vi "fpga_transmission_control_3V13.vi"() -> ()   [LabVIEW 2017]
uses:
  Control 1.ctl
  <vilib>/Platform/TimedLoop/XDataNode/timing_clust.ctl
  <vilib>/Platform/TimedLoop/XDataNode/nitl_modes.ctl
  <vilib>/Platform/TimedLoop/XDataNode/wakeup.ctl
  <vilib>/Instr/_visa.llb/VISA Configure Serial Port (Serial Instr).vi
  <vilib>/platform/TimedLoop/XDataNode/XDataNode.xnode
  <vilib>/Platform/TimedLoop/XDataNode/XDNodeRunTimeDep.lvlib
panel:
  out "Complete Time":u32
  out "Timer":u32
  out "Output":bool
  out "outcome":u32
  out "currentType":string
  out "Time":dbl(slide) scale=0.0..100.0
  out "Progress":dbl(slide) scale=0.0..100.0
  in  "error in (no error)":errorcluster
  out "PWM":bool
  out "pattern":u32
  in  "Timeslot":bool
  out "type":string
  out "Kombi Chart":cluster{u16, i16}(graph)
  out "contingency":string
  in  "Array":T2(array[cluster]) {"duration" step=1}
  out "Timeslot":i32
  out "Sign":bool
  out "deleted portion":u8[](array[numeric])
  out "data":bool
  out "x-y":u16
  out "Error String":string
  out "error out":errorcluster
  out "Timing":u32
  out "Int_pixel":i16
  out "Pixel":u16(graph)
  out "AD_Value":i16
  in  "millisecond timer value 2":u32
  out "AD_Chart":i16(graph)
  in  "Path":path
  out "Read":bool
  in  "Stop Program":bool
  in  "Start":bool
  in  "VISA resource name":refnum<visa-resource-name>
  # "UR Elektronik Biologie\nTerminal V 3.8"
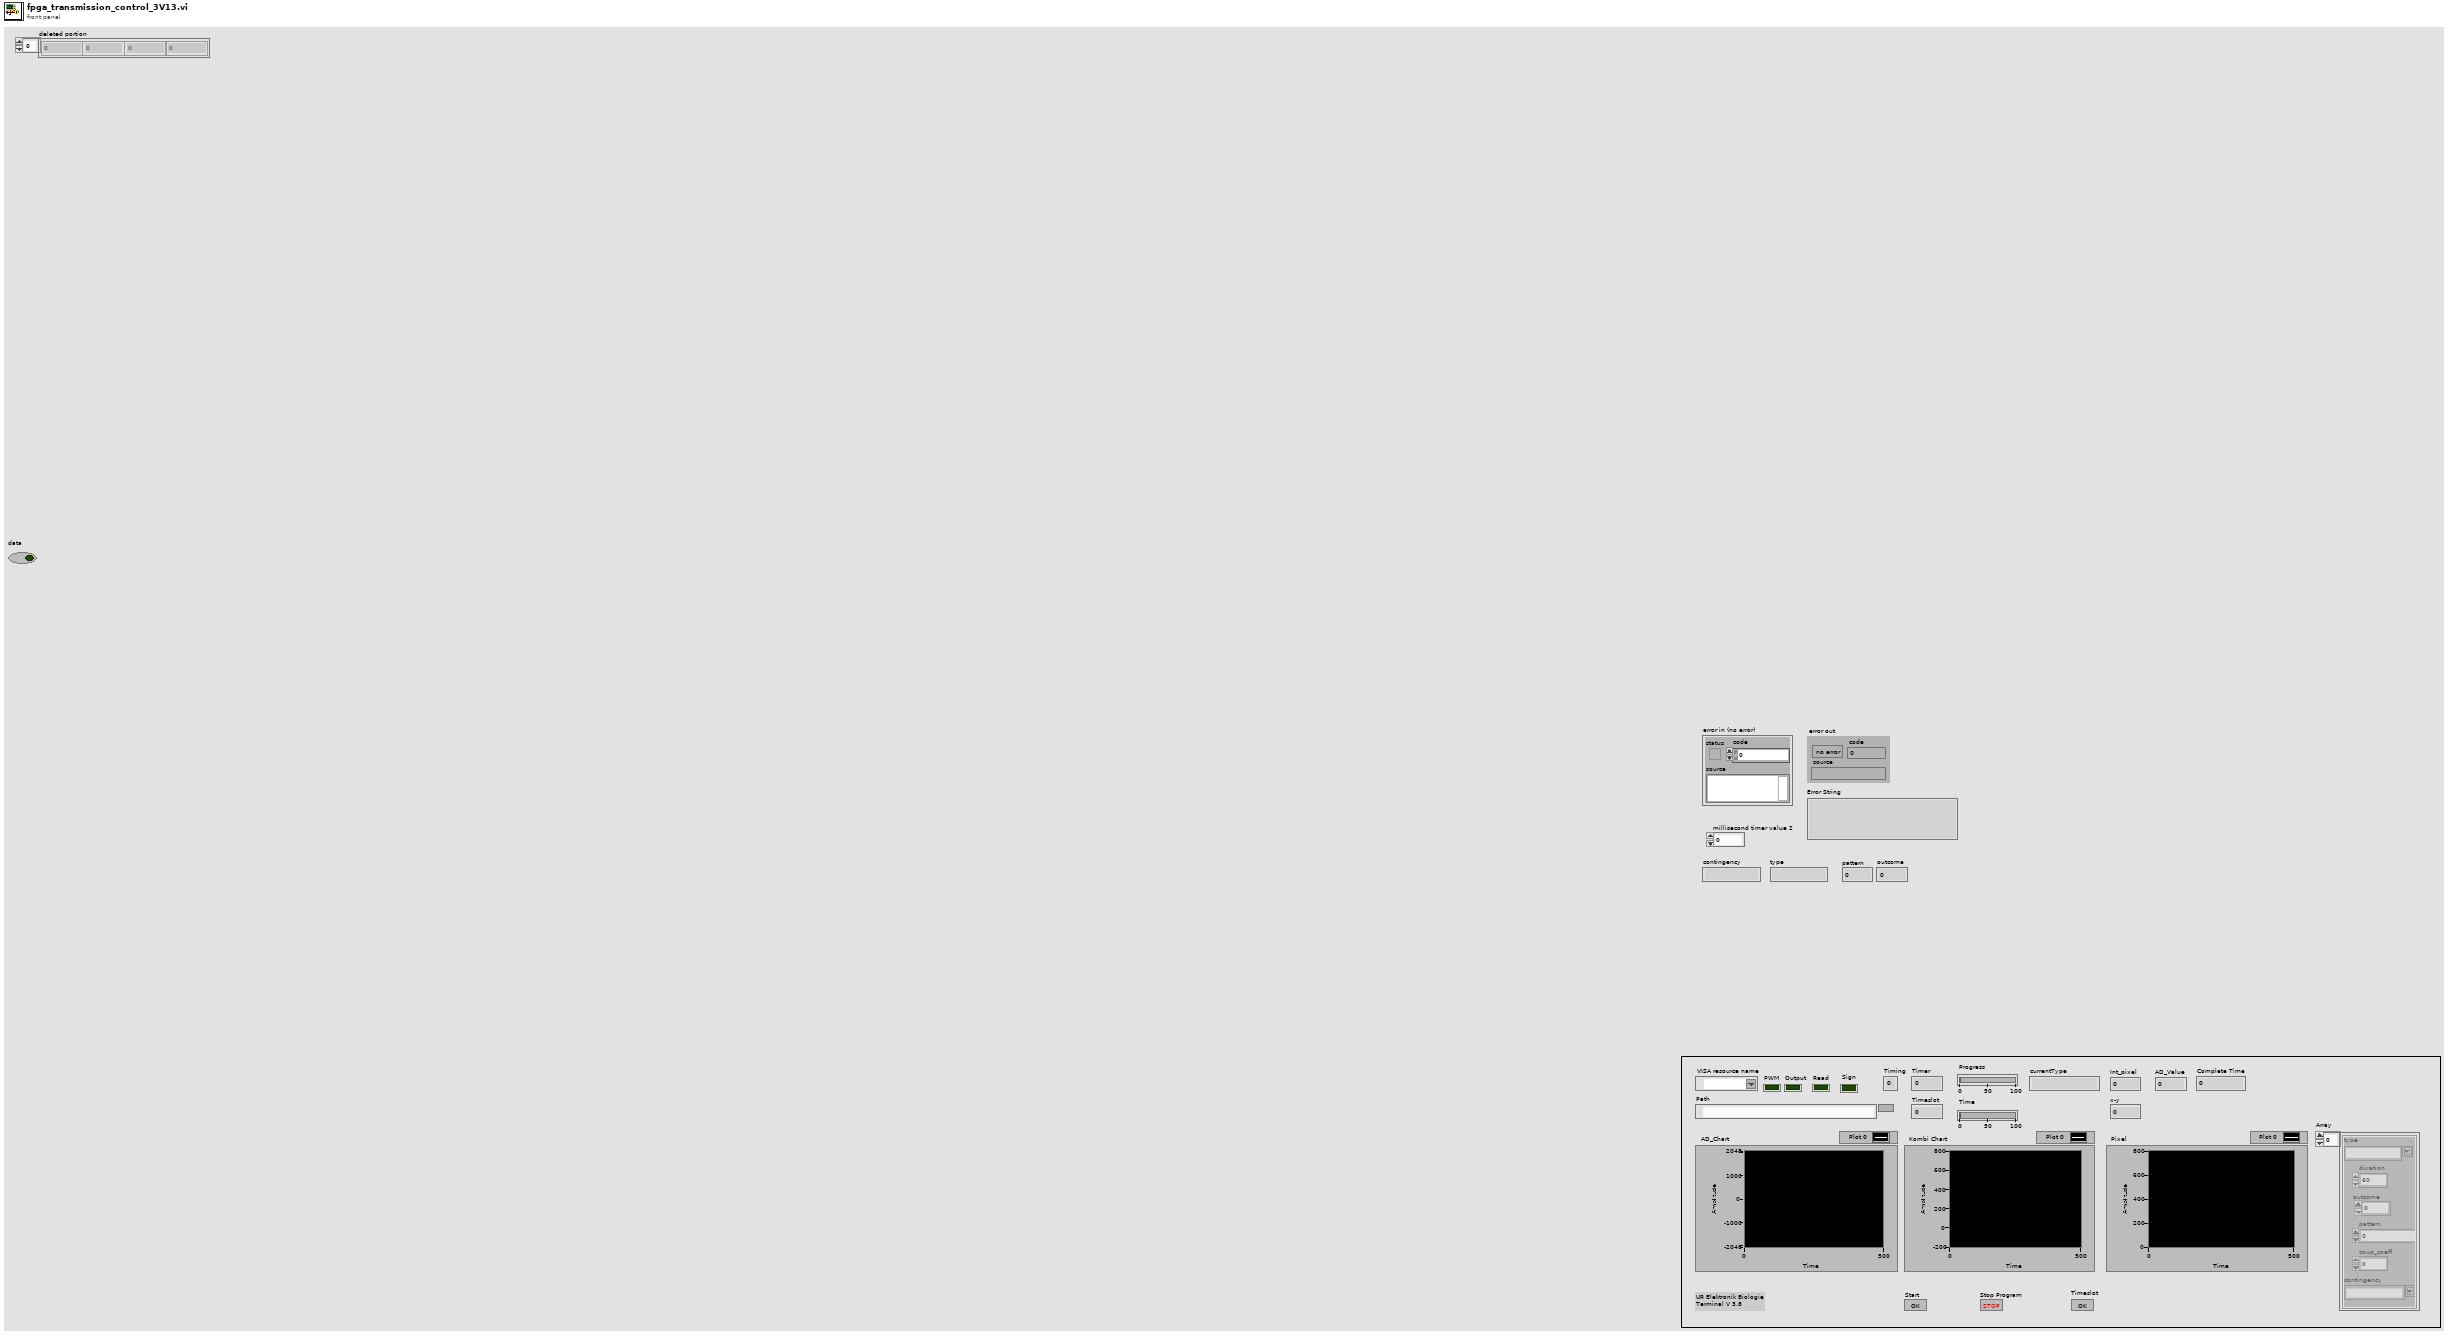
[diagram p1: front panel]
types:
  T1 = typedef "Control 1.ctl" = u32
  T2 = cluster{"type":string, "duration":T1, "outcome":u32, "pattern":u32, "coup_coeff":u32, "contingency":string}[]
  T3 = typedef "XDNodeRunTimeDep.lvlib/timing_clust.ctl" = cluster{"Expected End [f-1]":u64, "Actual End [f-1]":u64, "Finished Late? [f-1]":bool, "Expected End [i-1]":u64, "Actual End [i-1]":u64, "Finished Late? [i-1]":bool, "Expected Start [i]":u64, "Actual Start [i]":u64, "Expected Start [f]":u64, "Actual Start [f]":u64, "Source Name":string, "Structure Name":string, "Period":i64, "Deadline":i64, "Offset":i64, "Start":i64, "Priority":i32, "Timeout":i32, "Mode":T4, "Wakeup Reason":T5, "Error":errorcluster, "Source Type":string, "Secondary Source Type":string, "Global End Time":u64, "Global Start Time":u64, "Frame Duration":u64, "Iteration Duration":u64, "Assigned CPU":i32, "I/O Scan Engine Mode":u32}
  T4 = typedef "XDNodeRunTimeDep.lvlib/nitl_modes.ctl" = enum32{"No Change", "Process missed periods, maintain original phase", "Discard missed periods, maintain original phase", "Process missed periods, ignore original phase", "Discard missed periods, ignore original phase"}
  T5 = typedef "XDNodeRunTimeDep.lvlib/wakeup.ctl" = enum32{"Normal", "Aborted", "Asynchronous wakeup", "Timing source error", "Timed loop error", "Timeout"}
  T6 = cluster{"String":string, i32, i32, u32, u32, "String":string}[]
  T7 = cluster{"type":string, "duration":T1, "outcome":u32, "pattern":u32, "coup_coeff":u32, "contingency":string}
  T8 = enum16{"Idel", "State1", "State2", "State3", "State4"}
  T9 = enum16{"open", "replace", "create", "open or create", "replace or create", "replace or create with confirmation"}
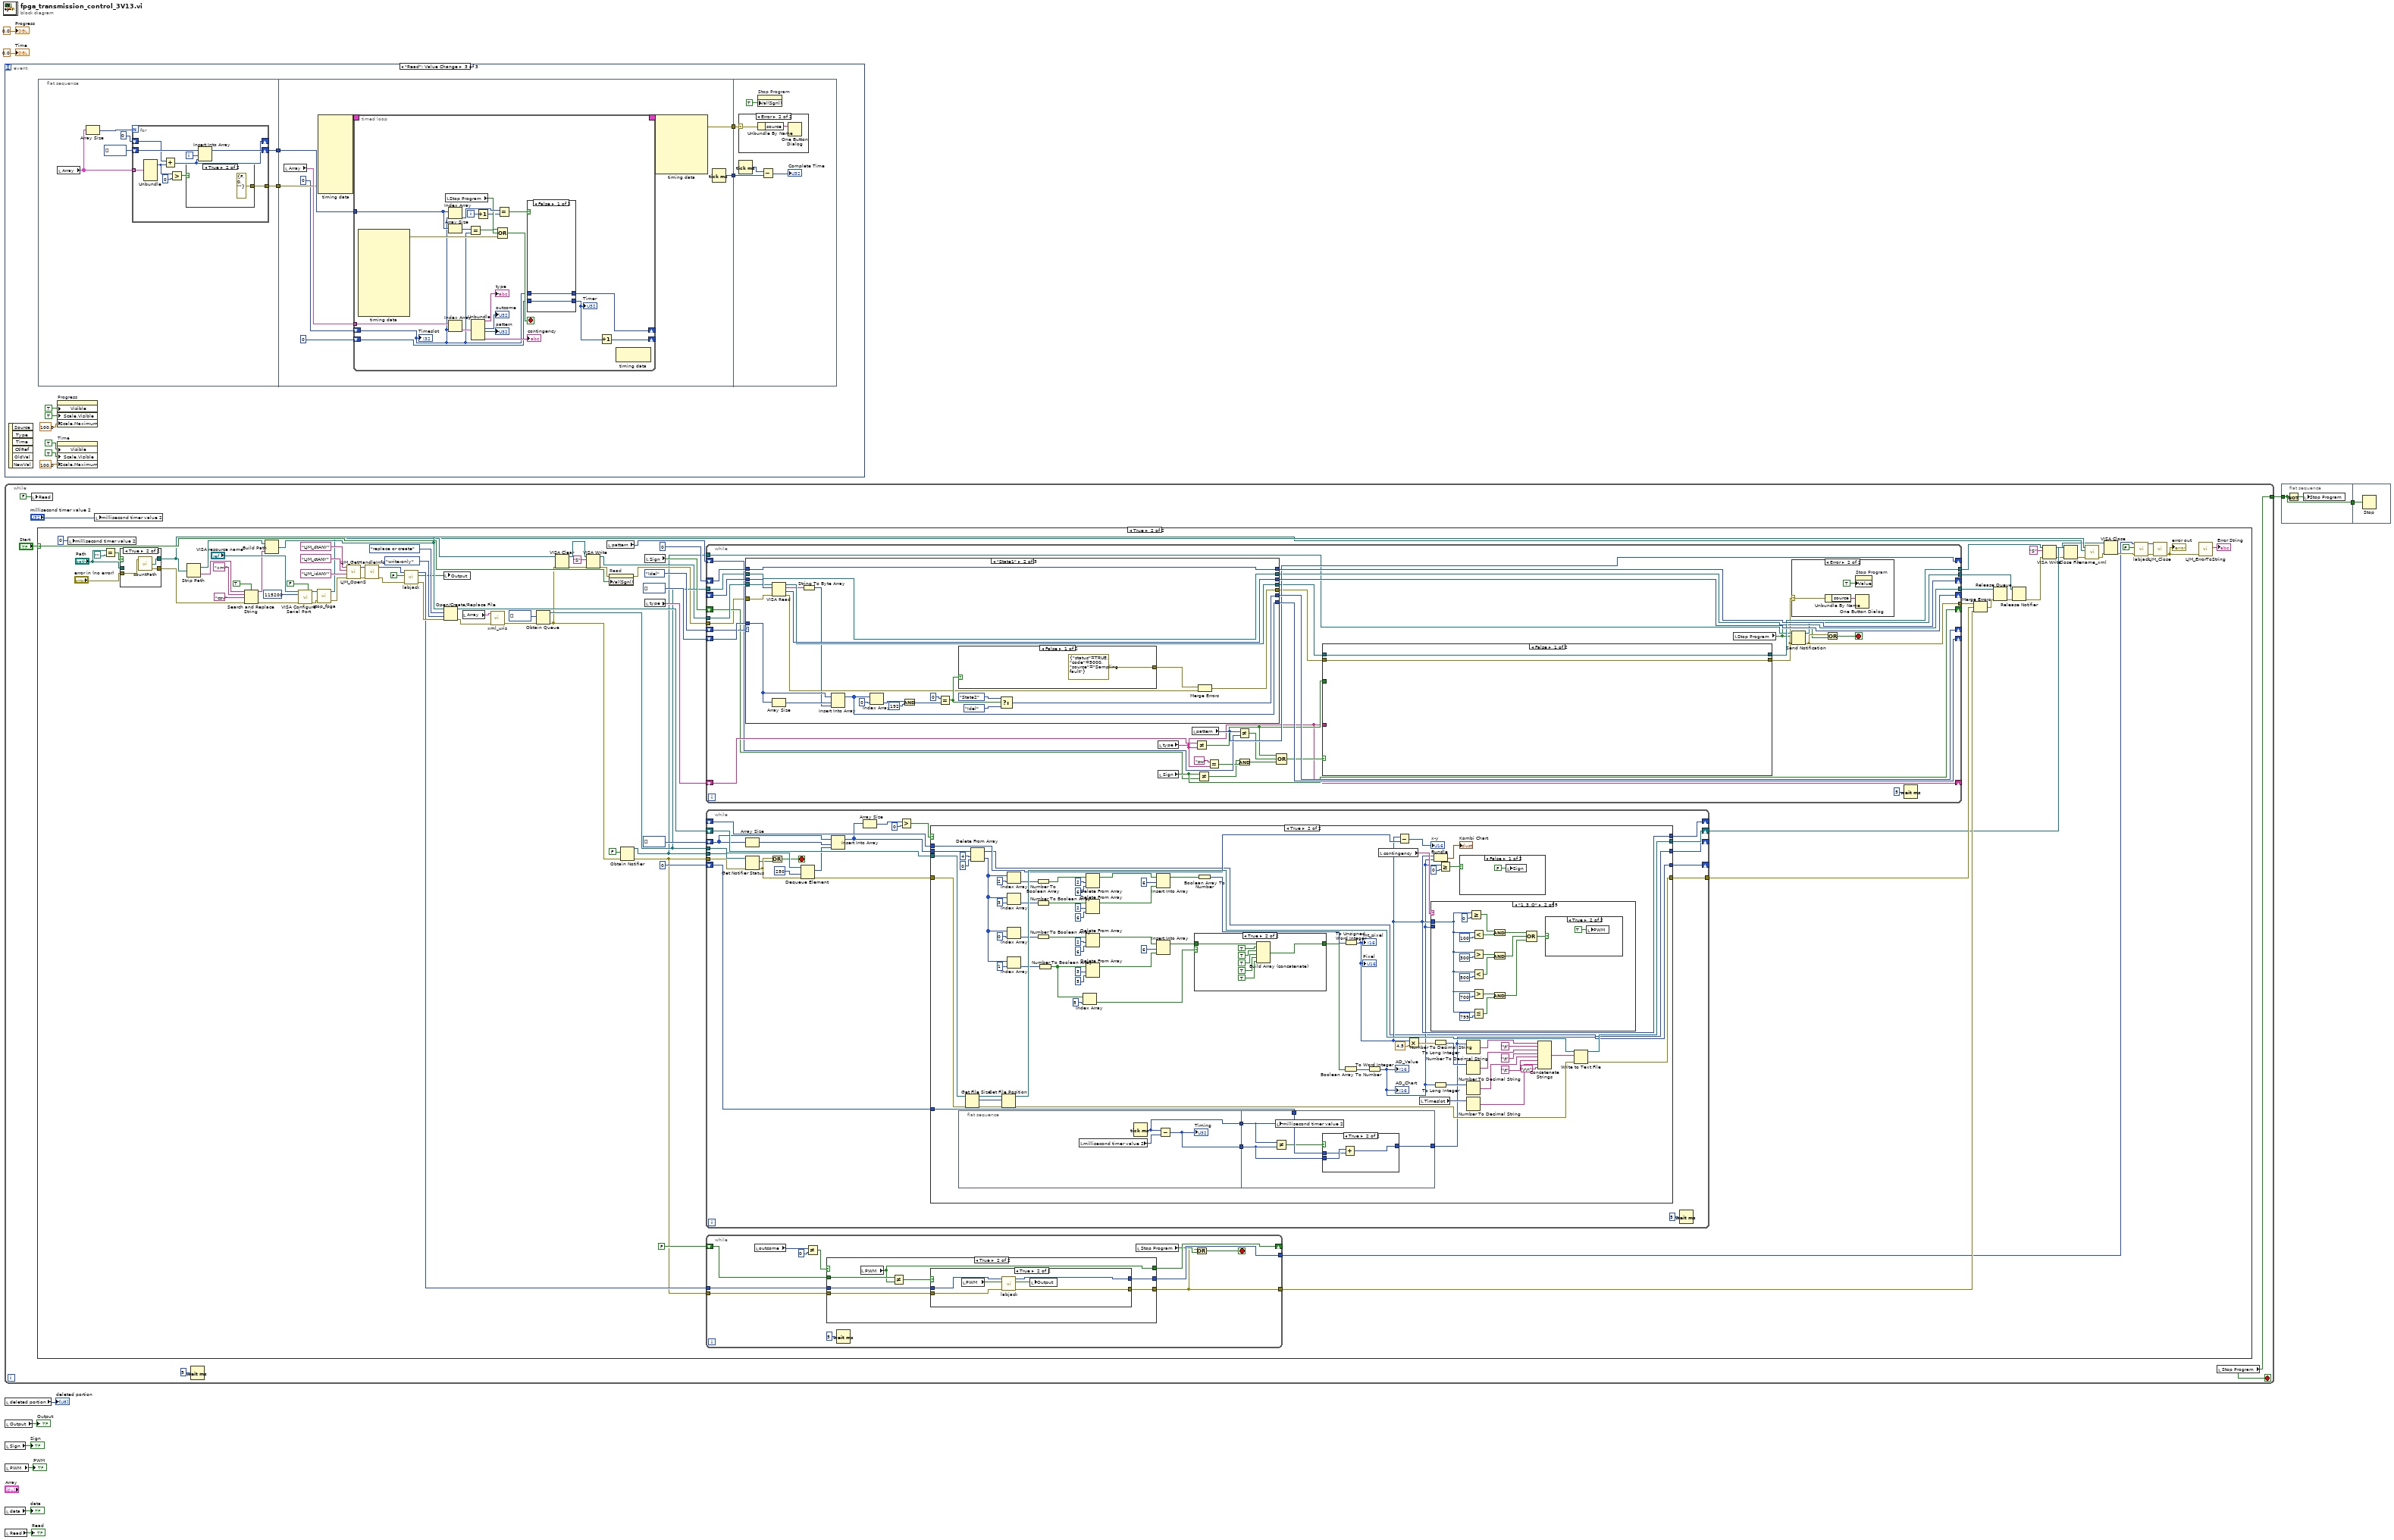
[diagram p0: block diagram]
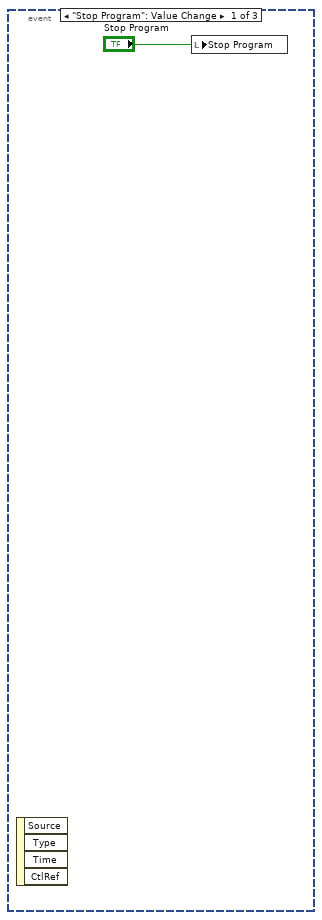
[diagram p2: hidden frame]
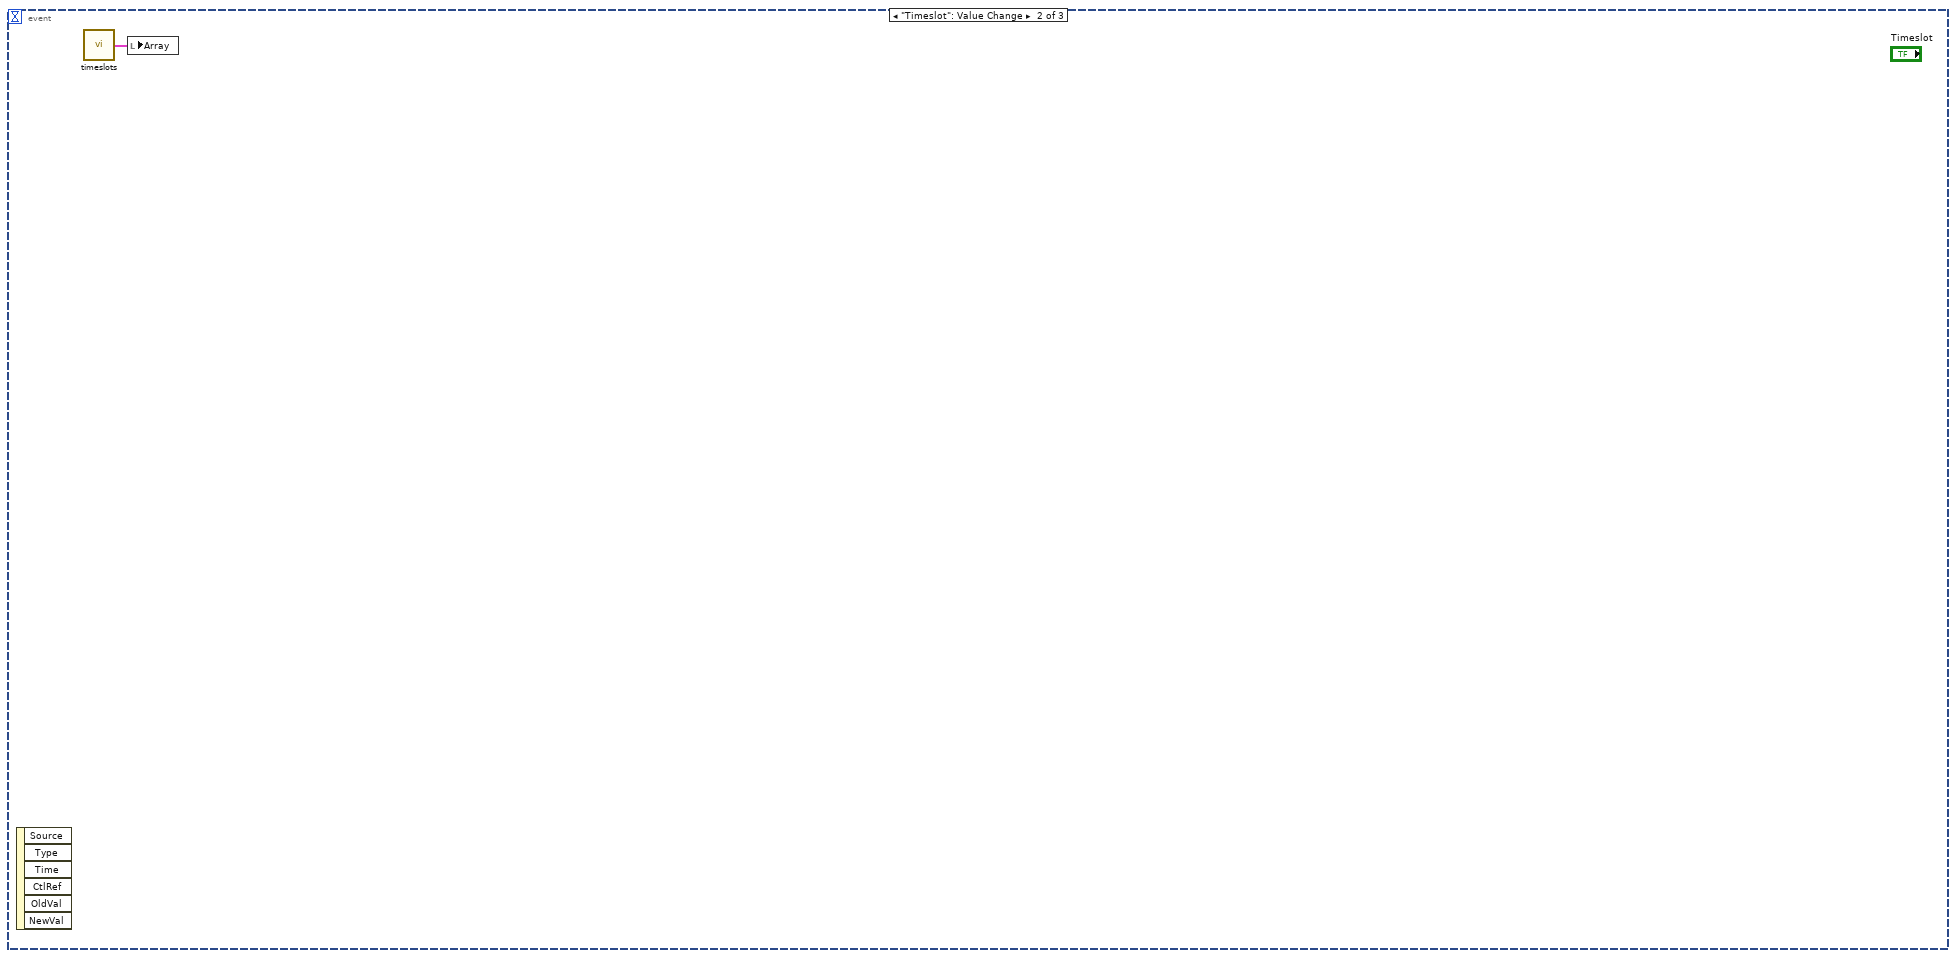
[diagram p3: hidden frame]
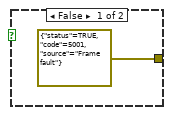
[diagram p4: hidden frame]
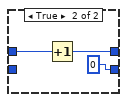
[diagram p5: hidden frame]
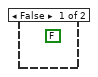
[diagram p7: hidden frame]
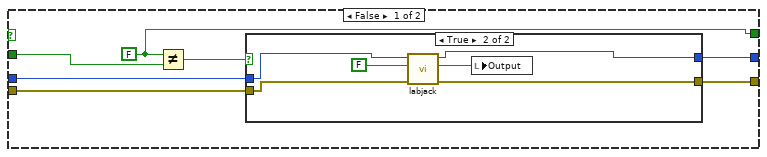
[diagram p9: hidden frame]
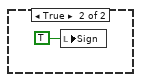
[diagram p13: hidden frame]
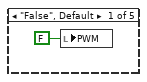
[diagram p14: hidden frame]
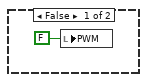
[diagram p15: hidden frame]
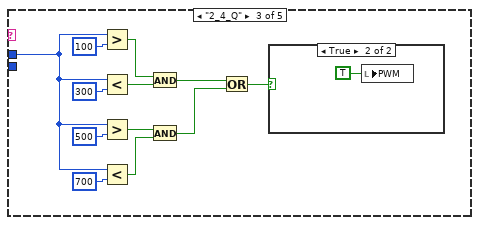
[diagram p16: hidden frame]
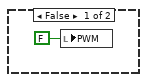
[diagram p17: hidden frame]
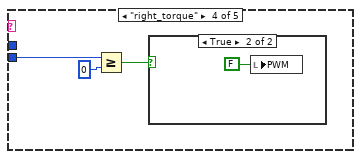
[diagram p18: hidden frame]
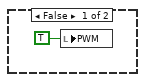
[diagram p19: hidden frame]
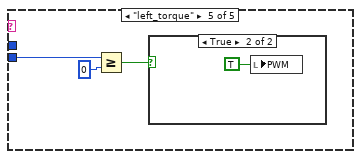
[diagram p20: hidden frame]
diagram:
  n1 = event shown="[2] \"Read\": Value Change" {
    selector: _ -> [_ _ _]
    dyn-events: _ -> [_ _ _]
    timeout: _ -> [_ _ _]
    event "Stop Program": Value Change {
      n2 = event-data() -> ()  [unwired: 1 in, 4 out]
      n3 = local write "Stop Program"("Stop Program") -> ()
    }
    event "Timeslot": Value Change {
      n4 = event-data() -> ()  [unwired: 1 in, 6 out]
      n5 = call "timeslots.vi"() -> ("array of clusters"=w12:T6)  [unwired: 1 in, 1 out]
      n6 = local write "Array"(w12) -> ()
    }
    event "Read": Value Change {
      n7 = event-data() -> ()  [unwired: 1 in, 6 out]
      n8 = flat-sequence {
        tunnel: [w24] -> w16
        tunnel: [w23] -> w15
        tunnel: w16 -> [w46]
        tunnel: w15 -> [w45]
        tunnel: [w44] -> w14
        tunnel: [w42] -> w13
        tunnel: w14 -> [w87]
        tunnel: w13 -> [w84]
        frame #0 {
          n9 = local read "Array"() -> (w27:T2)
          n10 = Array Size(array=w27) -> (size(s)=w28:i32)
          n11 = for {
            N: w28 -> [_]
            tunnel: w27 -> [w38] mode=indexing
            shift-right: [w36] -> w24
            shift-left: T1[] [] -> [w35]
            shift-right: [w33] -> _
            shift-left: T1 0 ("duration") -> [w34]
            tunnel: [w29] -> w23
            i -> [w37]
            n12 = Unbundle(w38) -> ("duration"=w31:T1)  [unwired: 5 out]
            n13 = Add(x=w34, y=w31) -> (x+y=w33:T1)
            n14 = Greater?(x=w31, y=T1 0) -> (0:w32:bool)
            n15 = case shown="True" w32 {
              tunnel: [errorcluster {"status"=TRUE, "code"=5001, "source"="Frame fault"} ("error constant") errorcluster {"status"=FALSE, "code"=0, "source"=""} ("error constant")] -> w29
              frame False {
              }
              frame True {
              }
            }
            n16 = Insert Into Array(array=w35, index=w37, new element=w33) -> (w36:T1[])
          }
        }
        frame #1 {
          n17 = local read "Array"() -> (w47:T2)
          n18 = node-c288(w45) -> (w49:T3)  [unwired: 9 in]
          n19 = timed-loop {
            timing: w49 -> [_]
            timing-out: [_] -> w48
            tunnel: w47 -> [w65]
            tunnel: w46 -> [w59]
            shift-right: [w62] -> _
            shift-left: T1 0 ("duration") -> [w57]
            shift-right: [w52] -> _
            shift-left: 0 -> [w51]
            i -> [w54]
            stop <- w64 stop-if-true
            n20 = node-c288() -> (w63:errorcluster)  [unwired: 1 in, 11 out]
            n21 = local read "Stop Program"() -> (w56:bool)
            n22 = Index Array(array=w59, index=w57) -> (element=w61:T1)
            n23 = Array Size(array=w59) -> (size(s)=w58:i32)
            n24 = Index Array(array=w65, index=w57) -> (element=w70:T7)
            n25 = Equal?(x=w58, y=w57) -> (x = y?=w55:bool)
            n26 = Unbundle(w70) -> ("type"=→"type":string, "outcome"=→"outcome":u32, "pattern"=→"pattern":u32, "contingency"=→"contingency":string)  [unwired: 2 out]
            n27 = Increment(x=w54) -> (x+1=w53:i32)
            n28 = Equal?(x=w61, y=w53) -> (x = y?=w60:bool)
            n29 = Compound Arithmetic op=OR(w56, w55, w63) -> (w64:bool)
            n30 = case shown="False" w60 {
              tunnel: [w72 w75] -> w62
              tunnel: w57 -> [w72 w74]
              tunnel: w51 -> [w71 _]
              tunnel: [w71 0] -> w50
              frame False {
              }
              frame True {
                n31 = Increment(x=w74) -> (x+1=w75:T1)
              }
            }
            "Timer" <- w50
            n32 = Increment(x=w50) -> (x+1=w52:i32)
            n33 = node-c288() -> ()  [unwired: 1 in, 1 out]
            "Timeslot" <- w57
          }
          n34 = node-c288(w48) -> (w44:errorcluster)  [unwired: 6 out]
          n35 = Tick Count (ms)() -> (millisecond timer value=w42:u32)
        }
        frame #2 {
          n36 = case shown="Error" w87 {
            selector: w87 -> [_ w90]
            frame No Error {
            }
            frame Error {
              n37 = Unbundle By Name(w90) -> ("source"=w89:string)
              n38 = One Button Dialog(message=w89) -> ()  [unwired: 1 in, 1 out]
            }
          }
          n39 = Tick Count (ms)() -> (millisecond timer value=w85:u32)
          n40 = property on="Stop Program" class="Bool (strict)"("Val(Sgnl)"=TRUE) -> ()  [unwired: 2 in, 2 out]
          n41 = Subtract(x=w85, y=w84) -> (x-y=→"Complete Time":u32)
        }
      }
      n42 = property on="Progress" class="Slide (strict)"("Visible"=TRUE, "Scale.Visible"=TRUE ("Visible"), "Scale.Maximum"=100.0 ("Scale.Range:Maximum")) -> ()  [unwired: 2 in, 2 out]
      n43 = property on="Time" class="Slide (strict)"("Visible"=TRUE, "Scale.Visible"=TRUE ("Visible"), "Scale.Maximum"=100.0 ("Scale.Range:Maximum")) -> ()  [unwired: 2 in, 2 out]
    }
  }
  n44 = while {
    tunnel: [w94] -> w10
    stop <- w94 stop-if-true
    n45 = local write "Read"(FALSE) -> ()
    n46 = case shown="True" "Start" {
      selector: "Start" -> [_ w172]
      frame False {
        (unwired) FALSE
      }
      frame True {
        n47 = local write "millisecond timer value 2"(u32 0 ("millisecond timer value 2")) -> ()
        n48 = Equal?(x="Path", y=path "") -> (x = y?=w159:bool)
        n49 = case shown="True" w159 {
          tunnel: [w180 w183] -> w125
          tunnel: "Path" -> [w180 _]
          tunnel: [w179 w182] -> w134
          tunnel: "error in (no error)" -> [w179 w181]
          frame False {
          }
          frame True {
            n50 = call "countPath.vi"("error in (no error)"=w181) -> ("error out"=w182:errorcluster, "appended path"=w183:path)
          }
        }
        n51 = Strip Path(path=w125) -> (stripped path=w138:path, name=w137:string)
        n52 = Search and Replace String(case sensitive?=TRUE ("ignore case? (F)"), input string=w137, search string="xml", replace string="csv" ("replace string (\"\")"), error in=w134) -> (result string=w131:string, error out=w133:errorcluster)  [unwired: 3 in, 2 out]
        n53 = Build Path(base path=w138, name or relative path=w131) -> (appended path=w126:path)
        n54 = call-poly "VISA Configure Serial Port"("VISA resource name"="VISA resource name", "Enable Termination\nChar (T)"=FALSE ("Enable Termination\nChar (T)"), "baud rate (9600)"=u32 115200, "error in (no error)"=w133) -> ("VISA resource name out"=w118:refnum<visa-resource-name>, "error out"=w117:errorcluster)  [unwired: 10 in]
        n55 = call "stop_fpga.vi"("error in (no error)"=w117, "reference"=w118) -> ("error out"=w116:errorcluster, "VISA resource name out"=w109:refnum<visa-resource-name>)  [unwired: 2 in]
        n56 = call "LJM_OpenS.vi"("error in"=w116, "Identifier"="LJM_idANY", "ConnectionType"="LJM_ctANY", "DeviceType"="LJM_dtANY") -> ("error out"=w162:errorcluster, "Handle"=w161:i32)  [unwired: 6 in]
        n57 = call "LJM_GetHandleInfo.vi"("error in"=w162, "Handle In"=w161) -> ("error out"=w164:errorcluster, "Handle Out"=w163:i32)  [unwired: 2 in, 6 out]
        n58 = call "labjack.vi"("error out"=w164, "Boolean"=FALSE, "Handle Out"=w163) -> ("error out 2"=w167:errorcluster, "Boolean 2"=w124:bool, "Handle Out 2"=w166:i32)  [unwired: 6 in]
        n59 = local write "Output"(w124) -> ()
        n60 = Open/Create/Replace File(file path (use dialog)=w126, error in=w167, operation (0:open)=T9."replace or create", access (0:read/write)=enum16{"read/write", "read-only", "write-only"}."write-only") -> (refnum out=w141:refnum<file>, error out=w139:errorcluster)  [unwired: 2 in, 1 out]
        n61 = local read "Array"() -> (w140:T2)
        n62 = call "xml_uris.vi"("error in"=w139, "Array"=w140) -> ("error out"=w110:errorcluster)  [unwired: 2 in, 2 out]
        n63 = Obtain Queue(element data type=u8[] [], error in (no error)=w110) -> (queue out=w112:refnum<queue>, error out=w97:errorcluster)  [unwired: 3 in, 1 out]
        n64 = VISA Clear(VISA resource name=w109, error in (no error)=w97) -> (VISA resource name out=w108:refnum<visa-resource-name>, error out=w106:errorcluster)
        n65 = VISA Write(VISA resource name=w108, write buffer="S", error in (no error)=w106) -> (VISA resource name out=w107:refnum<visa-resource-name>, error out=w115:errorcluster)  [unwired: 1 out]
        n66 = local read "pattern"() -> (w144:u32)
        n67 = property on="Read" class="Bool (strict)"(error in=w115, "Val(Sgnl)"=w172) -> (error out=w105:errorcluster)  [unwired: 1 in, 1 out]
        n68 = Obtain Notifier(notification data type=FALSE, error in (no error)=w97) -> (notifier out=w103:refnum<notifier>, error out=w96:errorcluster)  [unwired: 2 in, 1 out]
        n69 = local read "Sign"() -> (w143:bool)
        n70 = local read "type"() -> (w168:string)
        n71 = while {
          tunnel: w107 -> [w428]
          shift-right: [w422] -> _
          shift-left: u8[] [] -> [w427]
          tunnel: [w404] -> w121
          shift-right: [w426] -> _
          shift-left: T8."Idel" -> [w425]
          shift-right: [w424] -> _
          shift-left: _ -> [w423]
          shift-right: [w421] -> _
          shift-left: u8 0 -> [w420]
          shift-right: [w411] -> _
          shift-left: w168 -> [w419]
          shift-right: [w418] -> _
          shift-left: w144 -> [w417]
          shift-right: [w416] -> _
          shift-left: w143 -> [w415]
          tunnel: w112 -> [w403]
          tunnel: [w402] -> w111
          tunnel: w103 -> [w399]
          tunnel: w105 -> [w400]
          tunnel: [w396] -> w100
          tunnel: [w397] -> w101
          stop <- w394 stop-if-true
          n72 = case shown="\"State1\"" w425 {
            tunnel: w428 -> [w546 w573 w591]
            tunnel: w400 -> [w547 w574 w585]
            tunnel: w427 -> [w550 w576 w598]
            tunnel: [w554 w577 w591] -> w405
            tunnel: [w553 w562 w584] -> w406
            tunnel: [w555 w575 w594] -> w426
            tunnel: [w552 w578 w592] -> w424
            tunnel: w423 -> [_ w579 w592]
            tunnel: [w550 w572 w597] -> w422
            tunnel: [w549 w571 u8 0] -> w421
            tunnel: w420 -> [w549 w571 _]
            tunnel: w403 -> [w544 w565 w587]
            tunnel: [w544 w565 w586] -> w402
            frame "Idel", Default {
              n73 = local write "data"(FALSE ("data")) -> ()
              n74 = property class="Serial Instr"(reference=w546, error in=w547) -> (reference out=w554:refnum<visa-resource-name>, error out=w553:errorcluster, "Serial Settings:Number of Bytes at Serial Port"=w552:u32)
              n75 = Greater Or Equal?(x=w552, y=u8 4) -> (x >= y?=w545:bool)
              n76 = Select(t=T8."State1", s=w545, f=T8."Idel") -> (s? t:f=w555:T8)
            }
            frame "State1" {
              n77 = VISA Read(VISA resource name=w573, byte count=w579, error in (no error)=w574) -> (VISA resource name out=w577:refnum<visa-resource-name>, read buffer=w559:string, return count=w578:u32, error out=w560:errorcluster)
              n78 = Array Size(array=w576) -> (size(s)=w564:i32)
              n79 = String To Byte Array(string=w559) -> (unsigned byte array=w558:u8[])
              n80 = Insert Into Array(array=w576, index=w564, new element=w558) -> (w572:u8[])
              n81 = Index Array(array=w572, index=0) -> (element=w569:u8)
              n82 = And(x=w569, y=u8 192) -> (x .and. y?=w568:u8)
              n83 = Equal?(x=u8 0, y=w568) -> (x = y?=w561:bool)
              n84 = case shown="False" w561 {
                tunnel: [errorcluster {"status"=TRUE, "code"=5000, "source"="Sampling fault"} ("error constant") errorcluster {"status"=FALSE, "code"=0, "source"=""} ("error constant")] -> w563
                frame False {
                }
                frame True {
                }
              }
              n85 = Select(t=T8."State2", s=w561, f=T8."Idel") -> (s? t:f=w575:T8)
              n86 = Merge Errors(w563, w560) -> (w562:errorcluster)
            }
            frame "State2" {
              n87 = Delete From Array(array=w598, length=4, index=0) -> (deleted portion=w588:u8[], array with subset deleted=w597:u8[])
              n88 = Array Size(array=w597) -> (size(s)=w596:i32)
              n89 = Enqueue Element(queue=w587, element=w588, error in (no error)=w585) -> (queue out=w586:refnum<queue>, error out=w584:errorcluster)  [unwired: 1 in, 1 out]
              n90 = Greater Or Equal?(x=w596, y=4) -> (x >= y?=w589:bool)
              n91 = Select(t=T8."State2", s=w589, f=T8."Idel") -> (s? t:f=w594:T8)
            }
          }
          n92 = local read "type"() -> (w411:string)
          n93 = local read "Sign"() -> (w416:bool)
          n94 = local read "pattern"() -> (w418:u32)
          n95 = Not Equal?(x=w419, y=w411) -> (x != y?=w412:bool)
          n96 = Not Equal?(x=w416, y=w415) -> (x != y?=w408:bool)
          n97 = Equal?(x="sw", y=w411) -> (x = y?=w409:bool)
          n98 = Not Equal?(x=w418, y=w417) -> (x != y?=w414:bool)
          n99 = And(x=w408, y=w409) -> (x .and. y?=w407:bool)
          n100 = Compound Arithmetic op=OR(w412, w414, w407) -> (w413:bool)
          n101 = case shown="False" w413 {
            tunnel: w405 -> [w433 w437]
            tunnel: [w433 w440] -> w404
            tunnel: w406 -> [w432 w436]
            tunnel: [w432 w441] -> w398
            tunnel: w411 -> [_ w434]
            tunnel: w412 -> [_ w435]
            frame False {
            }
            frame True {
              n102 = case shown="True" w435 {
                tunnel: [w443 w449] -> w439
                tunnel: [w444 w448] -> w438
                tunnel: w437 -> [w444 w446]
                tunnel: w436 -> [w443 w445]
                frame False {
                }
                frame True {
                  n103 = VISA Write(VISA resource name=w446, write buffer="1W", error in (no error)=w445) -> (VISA resource name out=w448:refnum<visa-resource-name>, error out=w449:errorcluster)  [unwired: 1 out]
                }
              }
              n104 = case shown="\"fs\"" w434 {
                tunnel: w438 -> [w451 w458 w463 w471 w482 w519]
                tunnel: [w453 w457 w462 w465 w481 w518] -> w440
                tunnel: w439 -> [w450 w456 w461 w470 w484 w521]
                tunnel: [w452 w455 w460 w466 w483 w520] -> w442
                frame "False", Default {
                  n105 = VISA Write(VISA resource name=w451, write buffer="s4s", error in (no error)=w450) -> (VISA resource name out=w453:refnum<visa-resource-name>, error out=w452:errorcluster)  [unwired: 1 out]
                }
                frame "optomotorR" {
                  n106 = VISA Write(VISA resource name=w458, write buffer="s3r", error in (no error)=w456) -> (VISA resource name out=w457:refnum<visa-resource-name>, error out=w455:errorcluster)  [unwired: 1 out]
                }
                frame "optomotorL" {
                  n107 = VISA Write(VISA resource name=w463, write buffer="s3l", error in (no error)=w461) -> (VISA resource name out=w462:refnum<visa-resource-name>, error out=w460:errorcluster)  [unwired: 1 out]
                }
                frame "yt" {
                  n108 = local read "pattern"() -> (w469:u32)
                  n109 = VISA Write(VISA resource name=w471, write buffer="s1s", error in (no error)=w470) -> (VISA resource name out=w468:refnum<visa-resource-name>, error out=w467:errorcluster)  [unwired: 1 out]
                  n110 = case shown="9" w469 {
                    tunnel: w468 -> [w474 w478]
                    tunnel: w467 -> [w473 w477]
                    tunnel: [w473 w476] -> w466
                    tunnel: [w474 w475] -> w465
                    frame 0, Default {
                    }
                    frame 9 {
                      n111 = VISA Write(VISA resource name=w478, write buffer="D", error in (no error)=w477) -> (VISA resource name out=w475:refnum<visa-resource-name>, error out=w476:errorcluster)  [unwired: 1 out]
                    }
                  }
                }
                frame "sw" {
                  n112 = local read "pattern"() -> (w480:u32)
                  n113 = case shown="7" w480 {
                    tunnel: w484 -> [w485 w490 w506]
                    tunnel: [w485 w488 w505] -> w483
                    tunnel: w482 -> [w486 w491 w504]
                    tunnel: [w486 w489 w503] -> w481
                    frame 0, Default {
                    }
                    frame 8 {
                      n114 = local read "Sign"() -> (w487:bool)
                      n115 = case shown="False" w487 {
                        tunnel: w490 -> [w493 w500]
                        tunnel: [w492 w499] -> w488
                        tunnel: w491 -> [w495 w498]
                        tunnel: [w494 w497] -> w489
                        frame True {
                          n116 = VISA Write(VISA resource name=w495, write buffer="G", error in (no error)=w493) -> (VISA resource name out=w494:refnum<visa-resource-name>, error out=w492:errorcluster)  [unwired: 1 out]
                        }
                        frame False {
                          n117 = VISA Write(VISA resource name=w498, write buffer="B", error in (no error)=w500) -> (VISA resource name out=w497:refnum<visa-resource-name>, error out=w499:errorcluster)  [unwired: 1 out]
                        }
                      }
                    }
                    frame 7 {
                      n118 = local read "Sign"() -> (w502:bool)
                      n119 = case shown="True" w502 {
                        tunnel: w506 -> [w508 w515]
                        tunnel: [w507 w514] -> w505
                        tunnel: w504 -> [w510 w513]
                        tunnel: [w509 w512] -> w503
                        frame False {
                          n120 = VISA Write(VISA resource name=w510, write buffer="G", error in (no error)=w508) -> (VISA resource name out=w509:refnum<visa-resource-name>, error out=w507:errorcluster)  [unwired: 1 out]
                        }
                        frame True {
                          n121 = VISA Write(VISA resource name=w513, write buffer="B", error in (no error)=w515) -> (VISA resource name out=w512:refnum<visa-resource-name>, error out=w514:errorcluster)  [unwired: 1 out]
                        }
                      }
                    }
                  }
                }
                frame "fs" {
                  n122 = local read "pattern"() -> (w517:u32)
                  n123 = case shown="4" w517 {
                    tunnel: w521 -> [w522 w528 w533 w538 w543]
                    tunnel: [w522 w526 w531 w536 w541] -> w520
                    tunnel: w519 -> [w523 w527 w532 w537 w542]
                    tunnel: [w523 w525 w530 w535 w540] -> w518
                    frame 0, Default {
                    }
                    frame 3 {
                      n124 = VISA Write(VISA resource name=w527, write buffer="s3s", error in (no error)=w528) -> (VISA resource name out=w525:refnum<visa-resource-name>, error out=w526:errorcluster)  [unwired: 1 out]
                    }
                    frame 2 {
                      n125 = VISA Write(VISA resource name=w532, write buffer="s2s", error in (no error)=w533) -> (VISA resource name out=w530:refnum<visa-resource-name>, error out=w531:errorcluster)  [unwired: 1 out]
                    }
                    frame 1 {
                      n126 = VISA Write(VISA resource name=w537, write buffer="s1s", error in (no error)=w538) -> (VISA resource name out=w535:refnum<visa-resource-name>, error out=w536:errorcluster)  [unwired: 1 out]
                    }
                    frame 4 {
                      n127 = VISA Write(VISA resource name=w542, write buffer="s4s", error in (no error)=w543) -> (VISA resource name out=w540:refnum<visa-resource-name>, error out=w541:errorcluster)  [unwired: 1 out]
                    }
                  }
                }
              }
              n128 = feedback #1() -> (w441:errorcluster)  [unwired: 1 in]
              n129 = feedback-in #1(w442) -> ()
              "currentType" <- w434
            }
          }
          n130 = local read "Stop Program"() -> (w395:bool)
          n131 = case shown="Error" w398 {
            selector: w398 -> [_ w430]
            frame No Error {
            }
            frame Error {
              n132 = Unbundle By Name(w430) -> ("source"=w429:string)
              n133 = property on="Stop Program" class="Bool (strict)"("Value"=TRUE) -> ()  [unwired: 2 in, 2 out]
              n134 = One Button Dialog(message=w429) -> ()  [unwired: 1 in, 1 out]
            }
          }
          n135 = Send Notification(notification=w395, notifier=w399, error in (no error)=w398) -> (notifier out=w397:refnum<notifier>, error out=w396:errorcluster)
          n136 = Or(x=w396, y=w395) -> (x .or. y?=w394:bool)
          n137 = Wait (ms)(milliseconds to wait=u32 5) -> ()  [unwired: 1 out]
        }
        n138 = while {
          shift-right: [w248] -> w129
          shift-left: w141 -> [w249]
          shift-right: [w246] -> _
          shift-left: _ -> [w247]
          shift-right: [w244] -> _
          shift-left: u32 0 -> [w243]
          shift-right: [w240] -> _
          shift-left: u8[] [] -> [w241]
          tunnel: w112 -> [w229]
          tunnel: w103 -> [w232]
          tunnel: w96 -> [w231]
          tunnel: [w245] -> w130
          stop <- w228 stop-if-true
          n139 = Array Size(array=w241) -> (size(s)=w239:i32)
          n140 = Get Notifier Status(notifier=w232, error in (no error)=w231) -> (current notification=w226:bool, error out=w227:errorcluster)  [unwired: 3 out]
          n141 = Or(x=w227, y=w226) -> (x .or. y?=w228:bool)
          n142 = Dequeue Element(queue=w229, timeout in ms (-1)=250, error in (no error)=w227) -> (element=w236:u8[], error out=w233:errorcluster)  [unwired: 2 out]
          n143 = Insert Into Array(array=w241, index=w239, new element=w236) -> (w235:u8[])
          n144 = Array Size(array=w235) -> (size(s)=w234:i32)
          n145 = Greater?(x=w234, y=0) -> (0:w237:bool)
          n146 = case shown="True" w237 {
            tunnel: w233 -> [w254 w278]
            tunnel: [w254 w322] -> w245
            tunnel: w249 -> [w253 w284]
            tunnel: [w253 w321] -> w248
            tunnel: [w252 w261] -> w246
            tunnel: w247 -> [w252 w279]
            tunnel: [w251 w265] -> w244
            tunnel: w243 -> [w251 w266]
            tunnel: w235 -> [w250 w259]
            tunnel: [w250 w256] -> w240
            frame False {
            }
            frame True {
              n147 = flat-sequence {
                tunnel: [w383] -> w320
                tunnel: [w382] -> w267
                tunnel: w320 -> [w386]
                tunnel: w267 -> [w387]
                tunnel: [w389] -> w265
                tunnel: w266 -> [w388]
                frame #0 {
                  n148 = local read "millisecond timer value 2"() -> (w384:u32)
                  n149 = Tick Count (ms)() -> (millisecond timer value=w383:u32)
                  n150 = Subtract(x=w383, y=w384) -> (x-y=w382:u32)
                  "Timing" <- w382
                }
                frame #1 {
                  n151 = Not Equal?(x=w386, y=w387) -> (x != y?=w385:bool)
                  n152 = local write "millisecond timer value 2"(w386) -> ()
                  n153 = case shown="True" w385 {
                    tunnel: w387 -> [_ w393]
                    tunnel: [u32 0 w392] -> w389
                    tunnel: w388 -> [_ w391]
                    frame False {
                    }
                    frame True {
                      n154 = Add(x=w393, y=w391) -> (x+y=w392:u32)
                    }
                  }
                }
              }
              n155 = Get File Size(file=w284, error in=w278) -> (refnum out=w327:refnum<file>, size (in bytes)=w326:i64, 0:w325:errorcluster)
              n156 = Delete From Array(array=w259, length=4, index=0) -> (deleted portion=w255:u8[], array with subset deleted=w256:u8[])
              n157 = Set File Position(offset (in bytes) (0)=w326, refnum=w327, error in=w325) -> (refnum out=w323:refnum<file>, error out=w324:errorcluster)  [unwired: 1 in]
              n158 = Index Array(array=w255, index=2) -> (element=w281:u8)
              n159 = Index Array(array=w255, index=3) -> (element=w280:u8)
              n160 = Index Array(array=w255, index=0) -> (element=w283:u8)
              n161 = Index Array(array=w255, index=1) -> (element=w282:u8)
              n162 = Number To Boolean Array(number=w281) -> (Boolean array=w302:bool[])
              n163 = Number To Boolean Array(number=w280) -> (Boolean array=w305:bool[])
              n164 = Number To Boolean Array(number=w283) -> (Boolean array=w292:bool[])
              n165 = Number To Boolean Array(number=w282) -> (Boolean array=w311:bool[])
              n166 = Index Array(array=w311, index=5) -> (element=w313:bool)
              n167 = Delete From Array(array=w302, length=2, index=6 ("length")) -> (array with subset deleted=w315:bool[])  [unwired: 1 out]
              n168 = Delete From Array(array=w305, length=2, index=6) -> (array with subset deleted=w316:bool[])  [unwired: 1 out]
              n169 = Delete From Array(array=w292, length=2, index=6 ("length")) -> (array with subset deleted=w295:bool[])  [unwired: 1 out]
              n170 = Delete From Array(array=w311, length=3, index=5) -> (array with subset deleted=w300:bool[])  [unwired: 1 out]
              n171 = Insert Into Array(array=w315, index=6, new element=w316) -> (w309:bool[])
              n172 = Insert Into Array(array=w295, index=6, new element=w300) -> (w297:bool[])
              n173 = case shown="True" w313 {
                tunnel: w297 -> [w374 w381]
                tunnel: [w374 w376] -> w314
                frame False {
                }
                frame True {
                  n174 = Build Array (concatenate)(w381, TRUE ("new element/subarray"), TRUE ("new element/subarray"), TRUE ("new element/subarray"), TRUE ("new element/subarray"), TRUE ("element")) -> (w376:bool[])
                }
              }
              n175 = Boolean Array To Number(Boolean array=w309) -> (number=w310:u32)
              n176 = To Unsigned Word Integer(number=w310) -> (unsigned 16bit integer=w261:u16)
              "Pixel" <- w261
              "Int_pixel" <- w261
              n177 = Boolean Array To Number(Boolean array=w314) -> (number=w301:u32)
              n178 = To Word Integer(number=w301) -> (16bit integer=w260:i16)
              "AD_Chart" <- w260
              "AD_Value" <- w260
              n179 = local read "contingency"() -> (w268:string)
              n180 = Subtract(x=w261, y=w279) -> (x-y=→"x-y":u16)
              n181 = Multiply(x=w261, y=4.5) -> (x*y=w270:dbl)
              n182 = local read "Timeslot"() -> (w274:i32)
              n183 = case shown="\"1_3_Q\"" w268 {
                tunnel: w261 -> [_ w332 w358 _ _]
                tunnel: w260 -> [_ _ _ w364 w369]
                frame "False", Default {
                  n184 = local write "PWM"(FALSE ("pwm")) -> ()
                }
                frame "1_3_Q" {
                  n185 = Greater Or Equal?(x=w332, y=u16 0 ("x")) -> (x >= y?=w331:bool)
                  n186 = Less?(x=w332, y=u16 100) -> (x < y?=w342:bool)
                  n187 = Greater?(x=w332, y=u16 300 ("a")) -> (0:w344:bool)
                  n188 = Less?(x=w332, y=u16 500 ("b")) -> (x < y?=w343:bool)
                  n189 = Greater?(x=w332, y=u16 700) -> (0:w341:bool)
                  n190 = Less Or Equal?(x=w332, y=u16 799) -> (x <= y?=w339:bool)
                  n191 = And(x=w331, y=w342) -> (x .and. y?=w337:bool)
                  n192 = And(x=w344, y=w343) -> (x .and. y?=w336:bool)
                  n193 = And(x=w341, y=w339) -> (x .and. y?=w335:bool)
                  n194 = Compound Arithmetic op=OR(w337, w336, w335) -> (w334:bool)
                  n195 = case shown="True" w334 {
                    frame False {
                      n196 = local write "PWM"(FALSE ("pwm")) -> ()
                    }
                    frame True {
                      n197 = local write "PWM"(TRUE ("pwm")) -> ()
                    }
                  }
                }
                frame "2_4_Q" {
                  n198 = Greater?(x=w358, y=u16 100 ("x")) -> (0:w353:bool)
                  n199 = Less?(x=w358, y=u16 300) -> (x < y?=w354:bool)
                  n200 = Greater?(x=w358, y=u16 500 ("a")) -> (0:w357:bool)
                  n201 = Less?(x=w358, y=u16 700 ("b")) -> (x < y?=w355:bool)
                  n202 = And(x=w353, y=w354) -> (x .and. y?=w352:bool)
                  n203 = And(x=w357, y=w355) -> (x .and. y?=w356:bool)
                  n204 = Or(x=w352, y=w356) -> (x .or. y?=w351:bool)
                  n205 = case shown="True" w351 {
                    frame False {
                      n206 = local write "PWM"(FALSE ("pwm")) -> ()
                    }
                    frame True {
                      n207 = local write "PWM"(TRUE ("pwm")) -> ()
                    }
                  }
                }
                frame "right_torque" {
                  n208 = Greater Or Equal?(x=w364, y=i16 0) -> (x >= y?=w365:bool)
                  n209 = case shown="True" w365 {
                    frame False {
                      n210 = local write "PWM"(TRUE ("pwm")) -> ()
                    }
                    frame True {
                      n211 = local write "PWM"(FALSE ("pwm")) -> ()
                    }
                  }
                }
                frame "left_torque" {
                  n212 = Greater Or Equal?(x=w369, y=i16 0) -> (x >= y?=w370:bool)
                  n213 = case shown="True" w370 {
                    frame False {
                      n214 = local write "PWM"(FALSE ("pwm")) -> ()
                    }
                    frame True {
                      n215 = local write "PWM"(TRUE ("pwm")) -> ()
                    }
                  }
                }
              }
              n216 = To Long Integer(number=w270) -> (32bit integer=w269:i32)
              n217 = To Long Integer(number=w260) -> (32bit integer=w272:i32)
              n218 = Bundle(w261, w260) -> (→"Kombi Chart":cluster{u16, i16})  [unwired: 1 in]
              n219 = Greater Or Equal?(x=w260, y=i16 0) -> (x >= y?=w262:bool)
              n220 = case shown="False" w262 {
                frame False {
                  n221 = local write "Sign"(FALSE) -> ()
                }
                frame True {
                  n222 = local write "Sign"(TRUE) -> ()
                }
              }
              n223 = Number To Decimal String(number=w265) -> (decimal integer string=w277:string)  [unwired: 1 in]
              n224 = Number To Decimal String(number=w269) -> (decimal integer string=w317:string)  [unwired: 1 in]
              n225 = Number To Decimal String(number=w272) -> (decimal integer string=w275:string)  [unwired: 1 in]
              n226 = Number To Decimal String(number=w274) -> (decimal integer string=w273:string)  [unwired: 1 in]
              n227 = Concatenate Strings(w277, "\t" ("string"), w317, "\t" ("string"), w275, "\t" ("string"), w273, "\r\n") -> (w285:string)
              n228 = Write to Text File(file (use dialog)=w323, text=w285, error in=w324) -> (refnum out=w321:refnum<file>, error out=w322:errorcluster)  [unwired: 1 in, 1 out]
            }
          }
          n229 = Wait (ms)(milliseconds to wait=u32 5) -> ()  [unwired: 1 out]
        }
        n230 = while {
          tunnel: w166 -> [w194]
          tunnel: w96 -> [w193]
          shift-right: [w191] -> _
          shift-left: FALSE ("pwm") -> [w195]
          tunnel: [w192] -> w148
          tunnel: [w184] -> w173
          stop <- w185 stop-if-true
          n231 = local read "outcome"() -> (w190:u32)
          n232 = Not Equal?(x=w190, y=u32 0) -> (x != y?=w188:bool)
          n233 = case shown="True" w188 {
            tunnel: w195 -> [w198 w217]
            tunnel: w194 -> [w202 w212]
            tunnel: w193 -> [w200 w213]
            tunnel: [w201 w216] -> w192
            tunnel: [w199 w215] -> w184
            tunnel: [w197 w214] -> w191
            frame False {
              w197 = FALSE ("Boolean")
              n234 = Not Equal?(x=w197, y=w198) -> (x != y?=w196:bool)
              n235 = case shown="True" w196 {
                tunnel: w202 -> [w204 w210]
                tunnel: [w204 w209] -> w201
                tunnel: w200 -> [w203 w208]
                tunnel: [w203 w207] -> w199
                frame False {
                }
                frame True {
                  n236 = call "labjack.vi"("error out"=w208, "Boolean"=FALSE, "Handle Out"=w210) -> ("error out 2"=w207:errorcluster, "Boolean 2"=w205:bool, "Handle Out 2"=w209:i32)  [unwired: 6 in]
                  n237 = local write "Output"(w205) -> ()
                }
              }
            }
            frame True {
              n238 = local read "PWM"() -> (w214:bool)
              n239 = Not Equal?(x=w217, y=w214) -> (x != y?=w211:bool)
              n240 = case shown="True" w211 {
                tunnel: w212 -> [w219 w225]
                tunnel: w213 -> [w218 w224]
                tunnel: [w219 w223] -> w216
                tunnel: [w218 w222] -> w215
                frame False {
                }
                frame True {
                  n241 = local read "PWM"() -> (w221:bool)
                  n242 = call "labjack.vi"("error out"=w224, "Boolean"=w221, "Handle Out"=w225) -> ("error out 2"=w222:errorcluster, "Boolean 2"=w220:bool, "Handle Out 2"=w223:i32)  [unwired: 6 in]
                  n243 = local write "Output"(w220) -> ()
                }
              }
            }
          }
          n244 = Wait (ms)(milliseconds to wait=u32 5) -> ()  [unwired: 1 out]
          n245 = local read "Stop Program"() -> (w186:bool)
          n246 = Or(x=w184, y=w186) -> (x .or. y?=w185:bool)
        }
        n247 = Merge Errors(w100, w130, w173) -> (w99:errorcluster)
        n248 = Release Queue(queue=w111, error in (no error)=w99) -> (error out=w102:errorcluster)  [unwired: 1 in, 2 out]
        n249 = Release Notifier(notifier=w101, error in (no error)=w102) -> (error out=w98:errorcluster)  [unwired: 1 in, 2 out]
        n250 = VISA Write(VISA resource name=w121, write buffer="S", error in (no error)=w98) -> (VISA resource name out=w120:refnum<visa-resource-name>, error out=w122:errorcluster)  [unwired: 1 out]
        n251 = Close File(refnum=w129, error in=w122) -> (error out=w128:errorcluster)  [unwired: 1 out]
        n252 = call "rename_xml.vi"("error in"=w128, "xml"=w125, "csv"=w126) -> ("error out"=w127:errorcluster)  [unwired: 4 in]
        n253 = VISA Close(VISA resource name=w120, error in (no error)=w127) -> (error out=w153:errorcluster)
        n254 = call "labjack.vi"("error out"=w153, "Boolean"=FALSE, "Handle Out"=w148) -> ("error out 2"=w154:errorcluster, "Handle Out 2"=w152:i32)  [unwired: 6 in, 1 out]
        n255 = call "LJM_Close.vi"("error in"=w154, "Handle"=w152) -> ("error out"=w151:errorcluster)  [unwired: 9 in]
        "error out" <- w151
        n256 = call "LJM_ErrorToString.vi"("error in"=w151) -> ("String"=→"Error String":string)  [unwired: 10 in]
      }
    }
    n257 = local write "millisecond timer value 2"("millisecond timer value 2") -> ()
    n258 = Wait (ms)(milliseconds to wait=u32 5) -> ()  [unwired: 1 out]
    n259 = local read "Stop Program"() -> (w94:bool)
  }
  n260 = local read "deleted portion"() -> (→"deleted portion":u8[])
  n261 = local read "Output"() -> (→"Output":bool)
  n262 = local read "Sign"() -> (→"Sign":bool)
  n263 = local read "PWM"() -> (→"PWM":bool)
  n264 = local read "data"() -> (→"data":bool)
  n265 = local read "Read"() -> (→"Read":bool)
  n266 = flat-sequence {
    tunnel: w10 -> [w603]
    tunnel: [w603] -> w9
    tunnel: w9 -> [w604]
    frame #0 {
      n267 = Not(x=w603) -> (.not. x?=w602:bool)
      n268 = local write "Stop Program"(w602) -> ()
    }
    frame #1 {
      n269 = Stop(stop? (T)=w604) -> ()
    }
  }
  "Progress" <- 0.0 ("Slide")
  "Time" <- 0.0 ("Progress 2")
